vi "IS_EXE.vi"(3 "error in":errorcluster) -> (0 "error out":errorcluster, 1 "1 - EXE":bool)   [LabVIEW 2018]
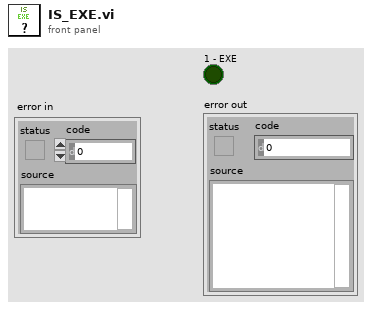
[diagram p1: front panel]
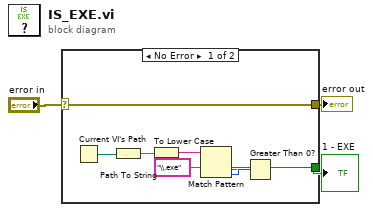
[diagram p0: block diagram]
diagram:
  n1 = case shown="No Error" "error in" {
    selector: "error in" -> [w4 w11]
    tunnel: [w5 _] -> w2
    tunnel: [w4 w11] -> w1
    frame No Error {
      n2 = Current VI's Path() -> (path=w10:path)
      n3 = Path To String(path=w10) -> (string=w9:string)
      n4 = To Lower Case(string=w9) -> (all lower case string=w8:string)
      n5 = Match Pattern(string=w8, regular expression="\\.exe") -> (offset past match=w6:i32)  [unwired: 1 in, 3 out]
      n6 = Greater Than 0?(x=w6) -> (x > 0?=w5:bool)
    }
    frame Error {
    }
  }
  "error out" <- w1
  "1 - EXE" <- w2
